vi "RVC 6-link serial robot.vi"() -> ()   [LabVIEW 2013]
uses:
  <vilib>/robotics/Kinematics/Robot/Robot Pose.ctl
  <vilib>/robotics/Kinematics/Analytical/Initialize Generic Serial Arm.vi
  <vilib>/robotics/Kinematics/Analytical/NI_Robotics_AnalyticKinematics.lvlib
  <vilib>/robotics/Kinematics/Robot/NI_Robotics_Serial Robot Arm.lvclass
  <vilib>/robotics/Kinematics/Link/Joint Type.ctl
  <vilib>/robotics/Kinematics/Link/NI_Robotics_Link.lvclass
panel:
  out "transformation":picture
  in  "Pose":u16(ring)=3 items=["qz", "qr", "qs", "qn"]
  in  "stop":bool
  out "3D Picture":refnum<vi>(3d-picture)
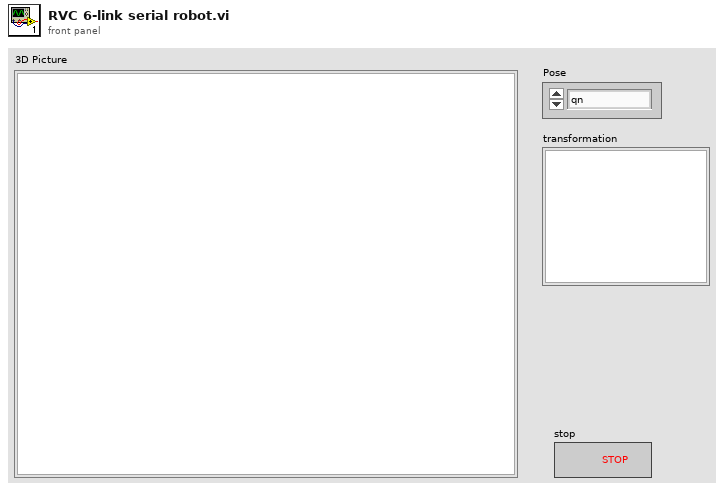
[diagram p1: front panel]
types:
  T1 = typedef "NI_Robotics_Serial Robot Arm.lvclass/Robot Pose.ctl" = cluster{"name":string, "description":string, "joint positions":dbl[]}
  T2 = typedef "NI_Robotics_Link.lvclass/Joint Type.ctl" = enum16{"Revolute", "Prismatic"}
  T3 = cluster{"Twist Angle":dbl, "Length":dbl, "Rotation Angle":dbl, "Offset Distance":dbl, "Joint Type":T2, "Joint Coordinate Offset":dbl}[]
  T4 = typedef "DH Kinematic Parameters.ctl" = cluster{"twist angle":dbl, "length":dbl, "rotation angle":dbl, "offset distance":dbl, "joint type":T2, "joint coordinate offset":dbl}
  T5 = typedef "NI_Matrix.lvlib/RealMatrix.ctl" = dbl[][]
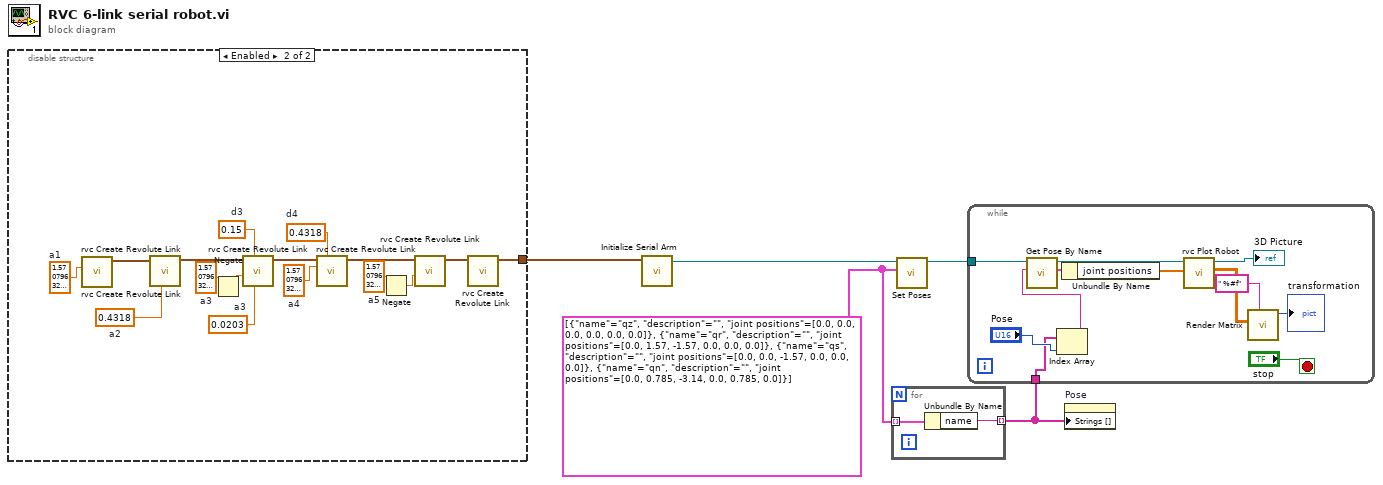
[diagram p0: block diagram]
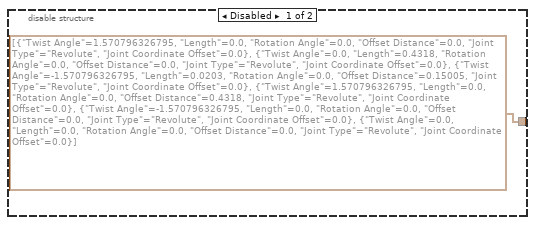
[diagram p2: hidden frame]
diagram:
  w2 = T1[] [{"name"="qz", "description"="", "joint positions"=[0.0, 0.0, 0.0, 0.0, 0.0, 0.0]}, {"name"="qr", "description"="", "joint positions"=[0.0, 1.57, -1.57, 0.0, 0.0, 0.0]}, {"name"="qs", "description"="", "joint positions"=[0.0, 0.0, -1.57, 0.0, 0.0, 0.0]}, {"name"="qn", "description"="", "joint positions"=[0.0, 0.785, -3.14, 0.0, 0.785, 0.0]}] ("serial arm poses")
  n1 = disable-structure shown="Enabled" {
    disable-tunnel: [T3 [{"Twist Angle"=1.570796326795, "Length"=0.0, "Rotation Angle"=0.0, "Offset Distance"=0.0, "Joint Type"=enum."Revolute", "Joint Coordinate Offset"=0.0}, {"Twist Angle"=0.0, "Length"=0.4318, "Rotation Angle"=0.0, "Offset Distance"=0.0, "Joint Type"=enum."Revolute", "Joint Coordinate Offset"=0.0}, {"Twist Angle"=-1.570796326795, "Length"=0.0203, "Rotation Angle"=0.0, "Offset Distance"=0.15005, "Joint Type"=enum."Revolute", "Joint Coordinate Offset"=0.0}, {"Twist Angle"=1.570796326795, "Length"=0.0, "Rotation Angle"=0.0, "Offset Distance"=0.4318, "Joint Type"=enum."Revolute", "Joint Coordinate Offset"=0.0}, {"Twist Angle"=-1.570796326795, "Length"=0.0, "Rotation Angle"=0.0, "Offset Distance"=0.0, "Joint Type"=enum."Revolute", "Joint Coordinate Offset"=0.0}, {"Twist Angle"=0.0, "Length"=0.0, "Rotation Angle"=0.0, "Offset Distance"=0.0, "Joint Type"=enum."Revolute", "Joint Coordinate Offset"=0.0}] w21] -> w5
    frame Disabled {
    }
    frame Enabled {
      w8 = 1.5707963267948966  # a5
      w9 = 0.4318  # d4
      w10 = 1.5707963267948966  # a4
      w12 = 1.5707963267948966  # a3
      w13 = 0.15  # d3
      w14 = 0.0203  # a3
      w18 = 0.4318  # a2
      w20 = 1.5707963267948966  # a1
      n2 = call "rvc Create Revolute Link.vi"("twist angle (alpha)"=w20) -> ("Array"=w19:T4[])  [unwired: 10 in]
      n3 = call "rvc Create Revolute Link.vi"("length (a)"=w18, "Array 2"=w19) -> ("Array"=w17:T4[])  [unwired: 9 in]
      n4 = Negate(x=w12) -> (-x=w11:dbl)
      n5 = call "rvc Create Revolute Link.vi"("length (a)"=w14, "offset distance (d)"=w13, "twist angle (alpha)"=w11, "Array 2"=w17) -> ("Array"=w16:T4[])  [unwired: 7 in]
      n6 = call "rvc Create Revolute Link.vi"("offset distance (d)"=w9, "twist angle (alpha)"=w10, "Array 2"=w16) -> ("Array"=w15:T4[])  [unwired: 8 in]
      n7 = Negate(x=w8) -> (-x=w7:dbl)
      n8 = call "rvc Create Revolute Link.vi"("twist angle (alpha)"=w7, "Array 2"=w15) -> ("Array"=w22:T4[])  [unwired: 9 in]
      n9 = call "rvc Create Revolute Link.vi"("Array 2"=w22) -> ("Array"=w21:T4[])  [unwired: 10 in]
    }
  }
  n10 = call-poly <vilib>:"Initialize Serial Arm.vi"("kinematic parameters"=w5) -> ("serial arm out"=w4:refnum<class "NI_Robotics_Serial Robot Arm.lvclass">)  [unwired: 9 in, 1 out]
  n11 = for {
    tunnel: w2 -> [w24] mode=indexing
    tunnel: [w23] -> w1 mode=indexing
    n12 = Unbundle By Name(w24) -> ("name"=w23:string)
  }
  n13 = call <vilib>:"Set Poses.vi"("serial arm poses"=w2, "serial arm in"=w4) -> ("serial arm out"=w3:refnum<class "NI_Robotics_Serial Robot Arm.lvclass">)  [unwired: 8 in, 1 out]
  n14 = while {
    tunnel: w3 -> [w33]
    tunnel: w1 -> [w29]
    stop <- "stop" stop-if-true
    n15 = Index Array(array=w29, index="Pose") -> (element=w28:string)
    n16 = call <vilib>:"Get Pose By Name.vi"("name"=w28, "serial arm in"=w33) -> ("serial arm pose"=w35:T1, "serial arm out"=w32:refnum<class "NI_Robotics_Serial Robot Arm.lvclass">)  [unwired: 7 in, 1 out]
    n17 = Unbundle By Name(w35) -> ("joint positions"=w34:dbl[])
    n18 = call "rvc Plot Robot.vi"("joint positions"=w34, "NI_Robotics_Serial Robot Arm in"=w32) -> ("forward kinematics"=w27:T5, "Scene Object Out"=→"3D Picture":refnum<vi>)  [unwired: 8 in]
    n19 = call "Render Matrix.vi"("format string"=" %#f", "A"=w27) -> ("picture out"=→"transformation":picture)  [unwired: 9 in]
  }
  n20 = property on="Pose" class="Ring (strict)"("Strings []"=w1) -> ()  [unwired: 2 in, 2 out]
